vi "Add WorksheetPart.vi"(8 "error in":errorcluster, 11 "SpreadsheetDoc in":refnum<k24>) -> (0 "error out":errorcluster, 2 "WorksheetPart":refnum<k24>, 3 "SpreadsheetDoc out":refnum<k24>)   [LabVIEW 2019, in "Open Xml.lvlib"]
uses:
  Open Xml.lvlib
  D:/git/Open-Xml-LabVIEW/Source/DocumentFormat.OpenXml.dll
  DocumentFormat.OpenXml.dll
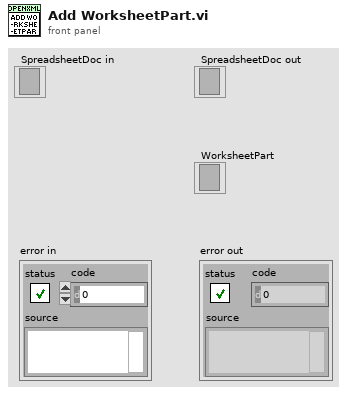
[diagram p1: front panel]
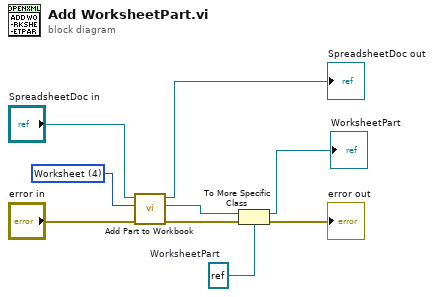
[diagram p0: block diagram]
diagram:
  w2 = refnum<k24> refnum  # WorksheetPart
  w5 = 4 items=["Connections", "PivotTableCacheDefinition", "PivotTableCacheRecords", "SharedString", "Worksheet", "WorkbookStyles"] ("PartType")
  n1 = call "Add Part to Workbook.vi"("error in"="error in", "PartType"=w5, "SpreadsheetDoc in"="SpreadsheetDoc in") -> ("error out"=w6:errorcluster, "OpenXmlPart"=w3:refnum<k24>, "SpreadsheetDoc out"=→"SpreadsheetDoc out":refnum<k24>)  [unwired: 6 in]
  n2 = To More Specific Class(target class=w2, reference=w3, error in=w6) -> (specific class reference=→"WorksheetPart":refnum<k24>, error out=→"error out":errorcluster)
